vi "kPID.vi"(8 "PID Gains":cluster{"Kp":dbl, "Kd":dbl, "Ki":dbl}, 10 "Position":dbl, 11 "Reference":dbl) -> (3 "Control":dbl)   [LabVIEW 2010, in "KevLib01.lvlib"]
uses:
  KevLib01.lvlib
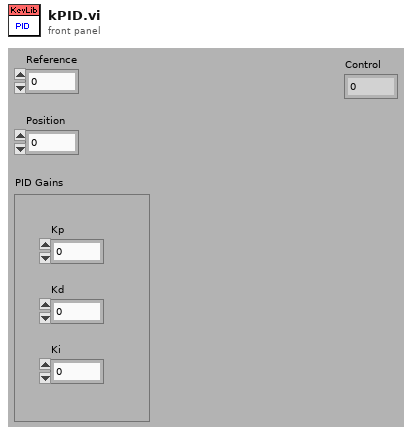
[diagram p1: front panel]
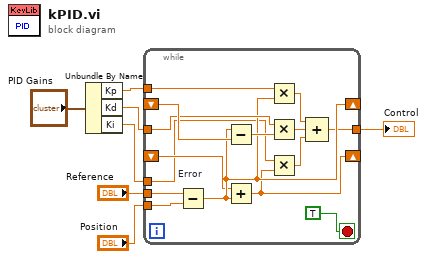
[diagram p0: block diagram]
diagram:
  n1 = Unbundle By Name("PID Gains") -> ("Kp"=w6:dbl, "Kd"=w3:dbl, "Ki"=w2:dbl)
  n2 = while {
    tunnel: w6 -> [w21]
    tunnel: "Reference" -> [w20]
    tunnel: "Position" -> [w19]
    shift-right: [w15] -> _
    shift-left: _ -> [w18]
    tunnel: w3 -> [w16]
    shift-right: [w13] -> _
    shift-left: _ -> [w14]
    tunnel: w2 -> [w12]
    tunnel: [w8] -> w1
    stop <- TRUE stop-if-true
    n3 = Subtract "Error"(x=w20, y=w19) -> (x-y=w15:dbl)
    n4 = Subtract(x=w15, y=w18) -> (x-y=w17:dbl)
    n5 = Add(x=w14, y=w15) -> (x+y=w13:dbl)
    n6 = Multiply(x=w21, y=w15) -> (x*y=w11:dbl)
    n7 = Multiply(x=w16, y=w17) -> (x*y=w10:dbl)
    n8 = Multiply(x=w12, y=w13) -> (x*y=w9:dbl)
    n9 = Compound Arithmetic op=ADD(w11, w10, w9) -> (w8:dbl)
  }
  "Control" <- w1
